vi "Control_Inst_DeInitDone.vi"(8 "error in (no error)":errorcluster, 11 "Cam_SLM_Controller in":refnum<class "Cam_SLM_Controller.lvclass">) -> (0 "error out":errorcluster, 3 "Cam_SLM_Controller out":refnum<class "Cam_SLM_Controller.lvclass">)   [LabVIEW 2023, in "Cam_SLM_controller.lvlib" / "Cam_SLM_Controller.lvclass"]
uses:
  Cam_SLM_Controller.lvclass
  Cam_SLM_Controller.lvclass/Cam_SLM_Controller.ctl
  <vilib>/ActorFramework/Stop Msg/Stop Msg.lvclass
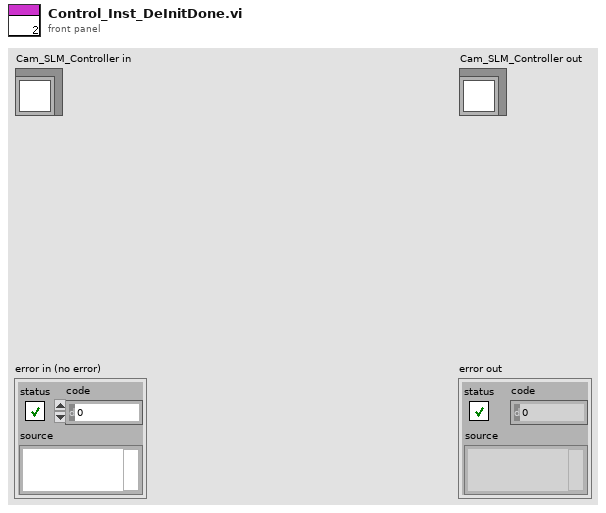
[diagram p1: front panel]
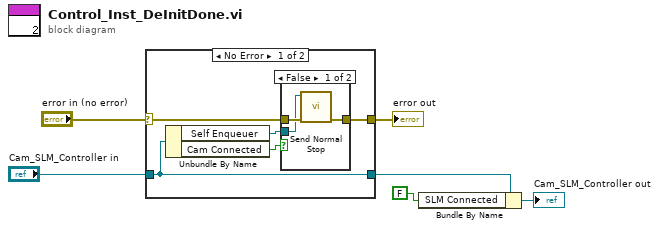
[diagram p0: block diagram]
diagram:
  n1 = case shown="No Error" "error in (no error)" {
    selector: "error in (no error)" -> [w9 w16]
    tunnel: "Cam_SLM_Controller in" -> [w8 w17]
    tunnel: [w10 w16] -> w1
    tunnel: [w8 w17] -> w3
    frame No Error {
      n2 = Unbundle By Name(w8) -> ("Self Enqueuer"=w7:refnum<class "Message Enqueuer.lvclass">, "Cam Connected"=w11:bool)
      n3 = case shown="False" w11 {
        tunnel: w9 -> [w14 w15]
        tunnel: [w13 w15] -> w10
        tunnel: w7 -> [w12 _]
        frame False {
          n4 = call <vilib>:"Send Normal Stop.vi"("error in (no error)"=w14, "Message Enqueuer"=w12) -> ("error out"=w13:errorcluster)  [unwired: 9 in]
        }
        frame True {
        }
      }
    }
    frame Error {
    }
  }
  "error out" <- w1
  n5 = Bundle By Name(cluster=w3, "SLM Connected"=FALSE ("Cam Connected")) -> (→"Cam_SLM_Controller out":refnum<class "Cam_SLM_Controller.lvclass">)
